vi "Vision_Processing_L_R10.vi"(0 "Current State":T1(ring)=enum."Normal - 5", 1 "Image Dst":T6=refnum, 2 "Inpute Image":T6=refnum, 3 "Startup Flag":bool, 5 "Current ROI Descriptor":T11={"Global Rectangle"=[22, 72, 300, 116], "Contours"=[{"ID"=enum."External", "Type"=12, "Coordinates"=[22, 72, 300, 116, 0]}]} {"Contours"."Type" items=["No Selection", "Point", "Line", "Rectangle", "Oval", "Polygon", "Freehand Region", "Annulus", "Unused2", "Unused3", "Broken Line", "Freehand Line", "Rotated Rectangle"]}, 6 "Avg Score - Last":dbl=954.6385864257812, 7 "error in (no error)":errorcluster, 8 "Current Settings":T9={"Curve Parameters"={"Extraction Mode"=1, "Edge Threshold"=150, "Edge Filter Size"=0, "Min Length"=15, "Row Search Step Size"=10, "Col Search Step Size"=10, "Max Endpoint Gap"=2, "Closed"=TRUE, "Subpixel"=TRUE}, "Match Mode"={"Rotation"=FALSE, "Scale"=TRUE, "Occlusion"=TRUE, "Reserved"=FALSE, "Reserved"=FALSE, "Reserved"=FALSE}, "Range Settings"=[{"Match Constraints"=0, "Min"=-2.0, "Max"=2.0}, {"Match Constraints"=1, "Min"=38.665856552124026, "Max"=79.77148170471192}, {"Match Constraints"=2, "Min"=0.0, "Max"=20.0}], "Number of Matches"=1, "Minimum Match Score"=879.6386, "SubPixel Accuracy"=TRUE, "Adv. Geometric Match Options 2"=[{"Setup Data Item"=20, "Item Value"=0.0}, {"Setup Data Item"=22, "Item Value"=1.0}]} {"Curve Parameters"."Extraction Mode" items=["Normal", "Uniform Regions"]; "Curve Parameters"."Edge Filter Size" items=["Fine", "Normal", "Contour Tracing"]; "Curve Parameters"."Max Endpoint Gap" min=0; "Curve Parameters"."Col Search Step Size" min=1 max=255 step=1; "Curve Parameters"."Row Search Step Size" min=1 max=255 step=1; "Curve Parameters"."Min Length" min=0; "Curve Parameters"."Edge Threshold" min=1 max=350 step=1; "Range Settings"."Max" format="%.2f"; "Range Settings"."Min" format="%.2f"; "Range Settings"."Match Constraints" items=["Rotation Angle (degrees)", "Scale Factor (%)", "Occlusion (%)"]; "Adv. Geometric Match Options 2"."Setup Data Item" items=["Curve Extraction Mode", "Curve Edge Threshold", "Curve Edge Filter Size", "Min Curve Length", "Curve Row Search Step Size", "Curve Col Search Step Size", "Curve Max Endpoint Gap", "Extract Closed Curves", "Enable Subpixel Curve Extraction", "Enable Correlation Score", "Enable Subpixel Accuracy", "Subpixel Iterations", "Subpixel Tolerance", "Initial Match List Length", "Enable Target Template Curve Score", "Min Match Separation Distance", "Min Match Separation Angle", "Min Match Separation Scale", "Max Match Overlap", "Enable Coarse Result", "Enable Calibration Support", "Enable Contrast Reversal", "Search Strategy", "Refinement Match Factor", "Subpixel Match Factor"]}, 9 "Sub Beacon Search Enable":bool[](array[boolean])=[FALSE, FALSE, FALSE, FALSE, FALSE], 10 "History Data - IN":T5={"Valid Beacon History - in"=[TRUE, TRUE, TRUE, TRUE, TRUE, TRUE, TRUE, TRUE, TRUE, TRUE, TRUE, TRUE, TRUE, TRUE, TRUE, TRUE, TRUE, TRUE, TRUE, TRUE], "Valid Score History"=[951.256103515625, 952.61669921875, 953.3775024414062, 959.8223266601562, 956.1203002929688, 952.1344604492188, 956.0997314453125, 948.7136840820312, 952.3104858398438, 956.33447265625, 949.6373291015625, 958.9732055664062, 951.8001708984375, 950.714599609375, 947.1436767578125, 952.746337890625, 992.2626342773438, 961.8504028320312, 971.9244384765625, 991.4178466796875], "Valid Scale History"=[59.26946258544922, 59.40597152709961, 59.318138122558594, 58.82406997680664, 59.27570343017578, 59.32193374633789, 59.52216339111328, 59.563385009765625, 59.49657440185547, 59.222198486328125, 59.44833755493164, 58.8350830078125, 59.57790756225586, 59.5397834777832, 59.55012512207031, 59.43376922607422, 59.040557861328125, 58.843505859375, 58.907012939453125, 58.86661911010742]} {"Valid Scale History" format="%#_13g"; "Valid Score History" format="%#_13g"}, 13 "Avg Scale - Last":dbl=59.21866912841797, 16 "History Size":i32=20) -> (11 "Avg Scale":dbl=59.21866912841797, 12 "Avg Score":dbl=954.6385864257812, 14 "Tracking Info 1":T2={"Tracking Coordinates"={"X"=160.85008239746094, "Y"=94.3125991821289}, "Current Valid"=TRUE, "Current State - Out"=enum."Normal - 5", "Setting Values"={"Min Scale"=38.67179412841797, "Max Scale"=79.78653259277344, "Min Score"=879.8142578125}}, 15 "Next Main ROI Descriptor":T3={"Global Rectangle"=[22, 72, 300, 116], "Contours"=[{"ID"=enum."External", "Type"=12, "Coordinates"=[22, 72, 300, 116, 0]}]} {"Contours"."Type" items=["No Selection", "Point", "Line", "Rectangle", "Oval", "Polygon", "Freehand Region", "Annulus", "Unused2", "Unused3", "Broken Line", "Freehand Line", "Rotated Rectangle"]}, 17 "Beacon - Scales":sgl[](array[numeric])=[0.0, 59.087868, 59.67315, 57.828133, 55.61106], 18 "History Data - Out":T4={"Valid Beacon History\nOut"=[TRUE, TRUE, TRUE, TRUE, TRUE, TRUE, TRUE, TRUE, TRUE, TRUE, TRUE, TRUE, TRUE, TRUE, TRUE, TRUE, TRUE, TRUE, TRUE, TRUE], "Valid Score History\nOut"=[951.256103515625, 952.61669921875, 953.3775024414062, 959.8223266601562, 956.1203002929688, 952.1344604492188, 956.0997314453125, 948.7136840820312, 952.3104858398438, 956.33447265625, 949.6373291015625, 958.9732055664062, 951.8001708984375, 950.714599609375, 947.1436767578125, 952.746337890625, 992.2626342773438, 961.8504028320312, 971.9244384765625, 991.4178466796875], "Valid Scale History\nOut"=[59.26946258544922, 59.40597152709961, 59.318138122558594, 58.82406997680664, 59.27570343017578, 59.32193374633789, 59.52216339111328, 59.563385009765625, 59.49657440185547, 59.222198486328125, 59.44833755493164, 58.8350830078125, 59.57790756225586, 59.5397834777832, 59.55012512207031, 59.43376922607422, 59.040557861328125, 58.843505859375, 58.907012939453125, 58.86661911010742]} {"Valid Scale History\nOut" format="%#_13g"; "Valid Score History\nOut" format="%#_13g"}, 19 "Y Coordinates":sgl[](array[numeric])=[0.0, 93.79849, 95.07948, 94.243286, 94.8068], 20 "Beacons Found":bool[](array[boolean])=[FALSE, TRUE, TRUE, TRUE, TRUE], 21 "X Coordinates":sgl[](array[numeric])=[0.0, 119.799255, 161.4642, 200.06786, 238.5652], 22 "Next State":T1(ring)=enum."Normal - 5", 23 "Lock Status":bool=TRUE, 24 "Startup Flag - out":bool, 25 "New Settings":T9={"Curve Parameters"={"Extraction Mode"=1, "Edge Threshold"=150, "Edge Filter Size"=0, "Min Length"=15, "Row Search Step Size"=10, "Col Search Step Size"=10, "Max Endpoint Gap"=2, "Closed"=TRUE, "Subpixel"=TRUE}, "Match Mode"={"Rotation"=FALSE, "Scale"=TRUE, "Occlusion"=TRUE, "Reserved"=FALSE, "Reserved"=FALSE, "Reserved"=FALSE}, "Range Settings"=[{"Match Constraints"=0, "Min"=-2.0, "Max"=2.0}, {"Match Constraints"=1, "Min"=38.665856552124026, "Max"=79.77148170471192}, {"Match Constraints"=2, "Min"=0.0, "Max"=20.0}], "Number of Matches"=1, "Minimum Match Score"=879.6386, "SubPixel Accuracy"=TRUE, "Adv. Geometric Match Options 2"=[{"Setup Data Item"=20, "Item Value"=0.0}, {"Setup Data Item"=22, "Item Value"=1.0}]} {"Curve Parameters"."Extraction Mode" items=["Normal", "Uniform Regions"]; "Curve Parameters"."Edge Filter Size" items=["Fine", "Normal", "Contour Tracing"]; "Curve Parameters"."Max Endpoint Gap" min=0; "Curve Parameters"."Col Search Step Size" min=1 max=255 step=1; "Curve Parameters"."Row Search Step Size" min=1 max=255 step=1; "Curve Parameters"."Min Length" min=0; "Curve Parameters"."Edge Threshold" min=1 max=350 step=1; "Range Settings"."Max" format="%.2f"; "Range Settings"."Min" format="%.2f"; "Range Settings"."Match Constraints" items=["Rotation Angle (degrees)", "Scale Factor (%)", "Occlusion (%)"]}, 27 "Right Image 2":T6(plugin-control))   [LabVIEW 2015]
uses:
  <vilib>/vision/Image Controls.llb/IMAQ Image.ctl
  <vilib>/vision/Pattern Matching.llb/IMAQ Curve Parameters.ctl
  <vilib>/vision/Pattern Matching.llb/IMAQ Match Range Setting.ctl
panel:
  in  "Current State 3":T1(ring)
  in  "Current State 2":T1(ring)
  in  "ROBOT STATE(fwd, bwd, neither)":i32
  out "beacon - Scores":sgl[](array[numeric])=[0.0, 997.01117, 999.39996, 999.517, 998.72253]
  in  "Minimum Score\nNormal 5":dbl=800.0
  in  "Minimum Score\nSub 4":dbl=850.0
  in  "Minimum Score\nSub 3":dbl=900.0
  in  "Minimum Score\nSub 2":dbl=950.0
  in  "Sub - 4 - FIle Path":path=path "/home/lvuser/natinst/bin/BeaconTemplates/4_beacons_left.png"
  in  "3 / 2\nTransition Scale":sgl=100.0
  in  "Score\nCushion- tight":dbl=75.0
  in  "Main ROI Decay\nper Fail (Vertical)":i32=5
  in  "ROI_factor(Horiztonal) (2 b)":sgl=1.5
  in  "ROI_factor(vertical) (2 b)":sgl=2.5
  in  "Sub - 2 File Path":path=path "/home/lvuser/natinst/bin/BeaconTemplates/2_beacons_left.png"
  out "Scale Decay \nFactor":dbl=20.552812576293945
  in  "Scale Decay \nFactor":dbl=5.0
  in  "Valid Treshold\nfor Lock":i16=3
  in  "Horiztonall Beacon \nCushion (pixels)":sgl=20.0
  out "New Min Score":dbl=879.6385864257812
  out "New Low Scale":dbl=38.665856552124026
  out "New high Scale":dbl=79.77148170471192
  in  "Absolute\nMinimum Score":dbl=800.0
  in  "Absolute\nMaximum Scale":dbl=300.0
  in  "Absolute\nMinimum Scale":dbl=10.0
  in  "Default No Lock\nSetting Values":T10={"Min Scale"=20.0, "Max Scale"=170.0, "Min Score"=800.0}
  in  "Score\nCushion":dbl=75.0
  out "Scale \nCushion":dbl=20.552812576293945
  in  "5 / 4\nTransition Scale":sgl=60.0
  in  "4 / 3\nTransition Scale":sgl=85.0
  in  "Timeout \nThrehsold":i32=1000
  in  "Main ROI Decay\nper Fail (Horiztonal)":i32=25
  in  "ROI_factor(Horiztonal) (4 b)":sgl=5.0
  in  "ROI_factor(vertical) (4 b)":sgl=1.5
  in  "ROI_factor(vertical) (5 b)":sgl=2.7
  in  "ROI_factor(Horiztonal) (5 b)":sgl=4.7
  out "Current  Score":sgl=951.2561
  out "Current  Scale":sgl=59.269463
  in  "Fail Count - In":i32
  in  "Sub Beacon Template File Path - ARRAY":path[](array[path])=[path "/home/lvuser/natinst/bin/BeaconTemplates/Sub1.png", path "/home/lvuser/natinst/bin/BeaconTemplates/Sub2.png", path "/home/lvuser/natinst/bin/BeaconTemplates/Sub3.png", path "/home/lvuser/natinst/bin/BeaconTemplates/Sub4.png", path "/home/lvuser/natinst/bin/BeaconTemplates/Sub5.png"]
  in  "Sub - 3 - FIle Path":path=path "/home/lvuser/natinst/bin/BeaconTemplates/3_beacons_left.png"
  in  "Normal - 5 - File Path":path=path "/home/lvuser/natinst/bin/BeaconTemplates/5_beacons.png"
  # "INPUTS"
  # "FILE PATHS"
  # "CONFIG"
  # "OUTPUTS"
  # "************"
  # "Range"
  # "Range"
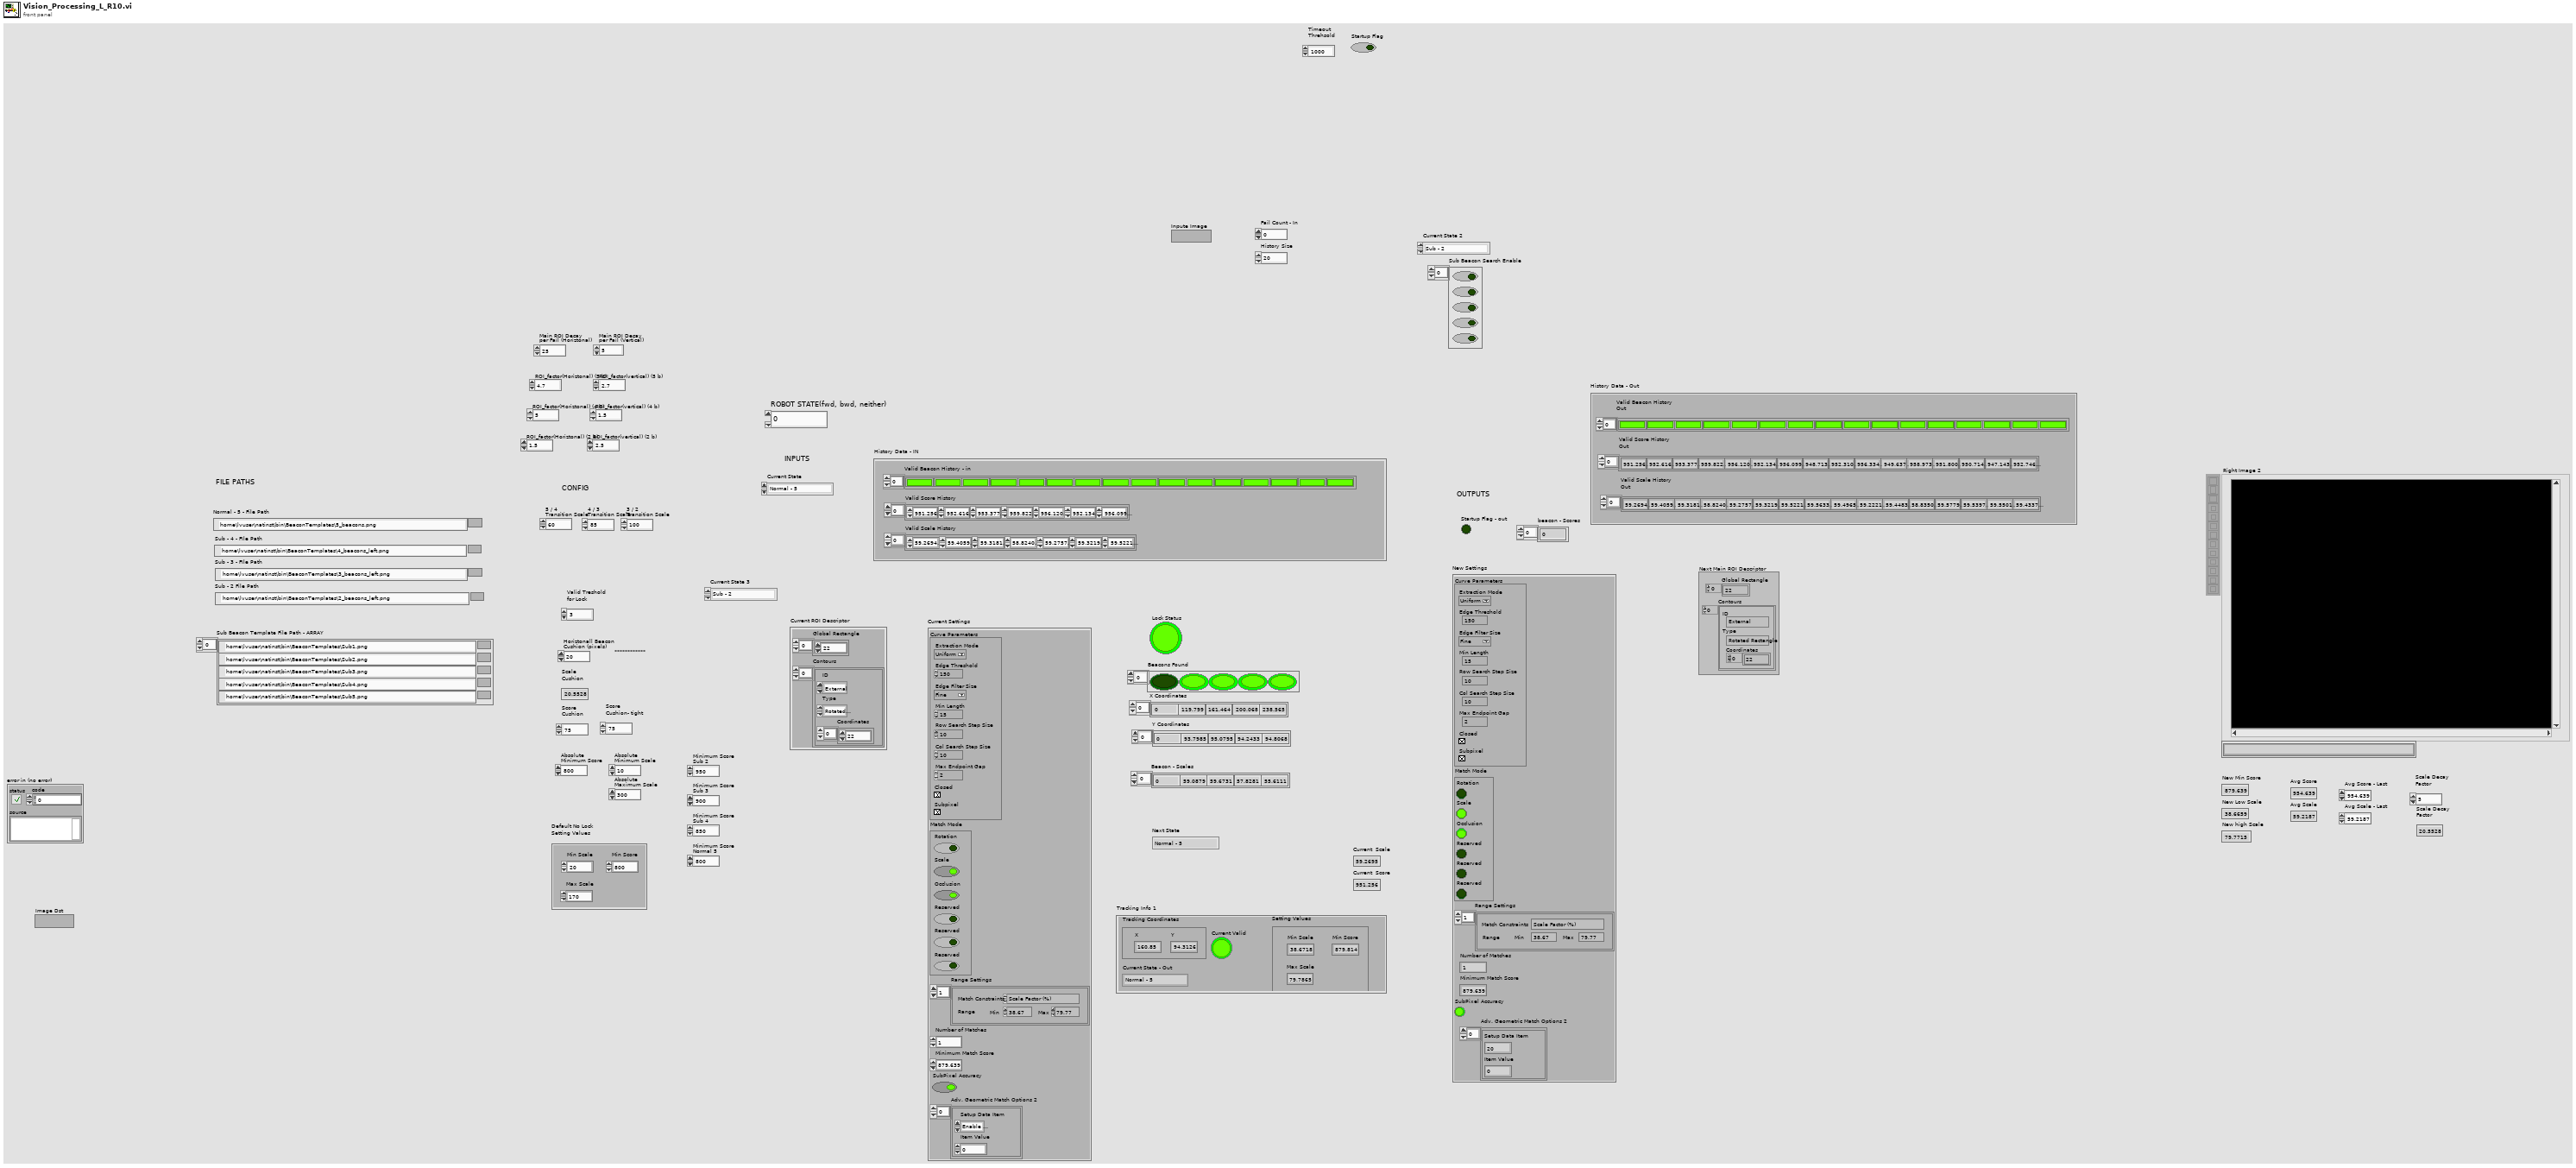
[diagram p1: front panel]
types:
  T1 = enum16{"Sub - 2", "Sub - 3", "Sub - 4", "Normal - 5"}
  T2 = cluster{"Tracking Coordinates":cluster{"X":dbl, "Y":dbl}, "Current Valid":bool, "Current State - Out":enum16{"Sub - 2", "Sub - 3", "Sub - 4", "Normal - 5"}, "Setting Values":cluster{"Min Scale":dbl, "Max Scale":dbl, "Min Score":dbl}}
  T3 = typedef "ROI Descriptor" = cluster{"Global Rectangle":i32[], "Contours":cluster{"ID":enum32{"External", "Internal"}, "Type":u32, "Coordinates":i32[]}[]}
  T4 = cluster{"Valid Beacon History\nOut":bool[], "Valid Score History\nOut":dbl[], "Valid Scale History\nOut":dbl[]}
  T5 = cluster{"Valid Beacon History - in":bool[], "Valid Score History":dbl[], "Valid Scale History":dbl[]}
  T6 = typedef "IMAQ Image.ctl" = refnum<image>
  T7 = typedef "IMAQ Curve Parameters.ctl" = cluster{"Extraction Mode":u32, "Edge Threshold":i32, "Edge Filter Size":u32, "Min Length":i32, "Row Search Step Size":i32, "Col Search Step Size":i32, "Max Endpoint Gap":i32, "Closed":bool, "Subpixel":bool}
  T8 = typedef "IMAQ Match Range Setting.ctl" = cluster{"Match Constraints":u32, "Min":dbl, "Max":dbl}
  T9 = cluster{"Curve Parameters":T7, "Match Mode":cluster{"Rotation":bool, "Scale":bool, "Occlusion":bool, "Reserved":bool, "Reserved":bool, "Reserved":bool}, "Range Settings":T8[], "Number of Matches":i32, "Minimum Match Score":sgl, "SubPixel Accuracy":bool, "Adv. Geometric Match Options 2":cluster{"Setup Data Item":u16, "Item Value":dbl}[]}
  T10 = cluster{"Min Scale":dbl, "Max Scale":dbl, "Min Score":dbl}
  T11 = cluster{"Global Rectangle":i32[], "Contours":cluster{"ID":enum32{"External", "Internal"}, "Type":u32, "Coordinates":i32[]}[]}
  T12 = typedef "IMAQ GM Match Report.ctl" = cluster{"Position":cluster{"x":sgl, "y":sgl}, "Angle":sgl, "Scale":sgl, "Score":sgl, "Bounding Box":cluster{"x":sgl, "y":sgl}[], "Contrast Reversed":bool, "Occlusion %":sgl, "Template Target Curve Score":sgl, "Target Template Curve Score":sgl, "Correlation Score":sgl}
  T13 = cluster{"Matches (Geometric Matching 1)[0]":T12, "Matches (Geometric Matching 1)[1]":T12, "Matches (Geometric Matching 1)[2]":T12, "Matches (Geometric Matching 1)[3]":T12, "Matches (Geometric Matching 1)[4]":T12, "Matches (Geometric Matching 1)[5]":T12, "Matches (Geometric Matching 1)[6]":T12, "Matches (Geometric Matching 1)[7]":T12, "Matches (Geometric Matching 1)[8]":T12}
  T14 = cluster{"Bounding Box[0]":cluster{"x":sgl, "y":sgl}, "Bounding Box[1]":cluster{"x":sgl, "y":sgl}, "Bounding Box[2]":cluster{"x":sgl, "y":sgl}, "Bounding Box[3]":cluster{"x":sgl, "y":sgl}, "Bounding Box[4]":cluster{"x":sgl, "y":sgl}, "Bounding Box[5]":cluster{"x":sgl, "y":sgl}, "Bounding Box[6]":cluster{"x":sgl, "y":sgl}, "Bounding Box[7]":cluster{"x":sgl, "y":sgl}, "Bounding Box[8]":cluster{"x":sgl, "y":sgl}}
  T15 = cluster{"index":u32, "Absolute\nMinimum Scale":dbl, "Absolute\nMaximum Scale":dbl}
  T16 = cluster{"New Low Scale":dbl, "New high Scale":dbl, "New Min Score":dbl}
  T17 = cluster{"Position":cluster{"x":sgl, "y":sgl}, bool, "Current State - Out":enum16{"Sub - 2", "Sub - 3", "Sub - 4", "Normal - 5"}, cluster{"New Low Scale":dbl, "New high Scale":dbl, "New Min Score":dbl}}
  T18 = cluster{"Position":cluster{"x":sgl, "y":sgl}, bool, "Current State":enum16{"Sub - 2", "Sub - 3", "Sub - 4", "Normal - 5"}, cluster{"New Low Scale":dbl, "New high Scale":dbl, "New Min Score":dbl}}
  T19 = typedef "IMAQ Rectangle" = cluster{"Left":i32, "Top":i32, "Right":i32, "Bottom":i32, "Rotation":dbl}
  T20 = cluster{"index":u32, "Min Scale":dbl, "Max Scale":dbl}
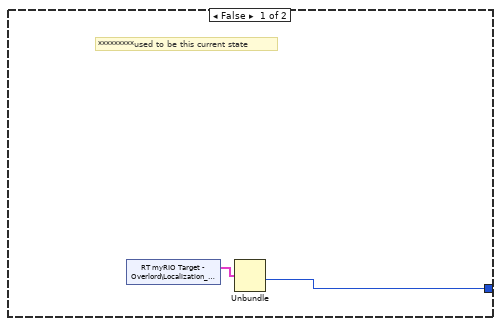
[diagram p4: hidden frame]
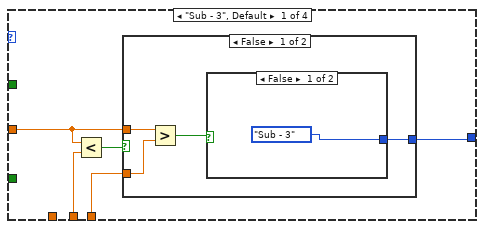
[diagram p5: hidden frame]
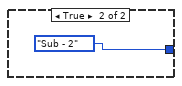
[diagram p6: hidden frame]
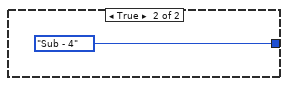
[diagram p7: hidden frame]
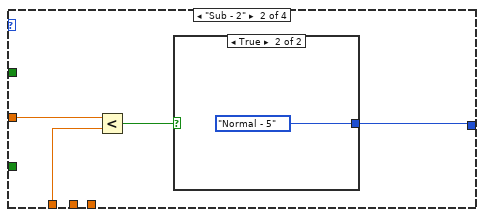
[diagram p8: hidden frame]
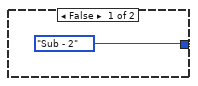
[diagram p9: hidden frame]
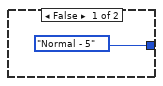
[diagram p10: hidden frame]
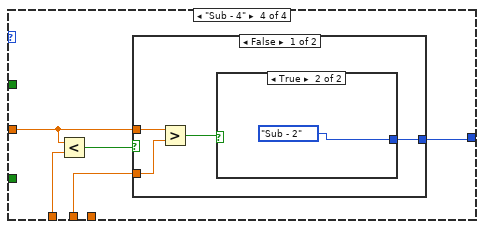
[diagram p11: hidden frame]
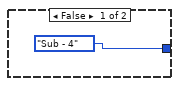
[diagram p12: hidden frame]
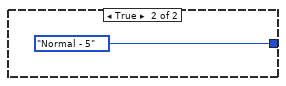
[diagram p13: hidden frame]
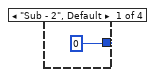
[diagram p15: hidden frame]
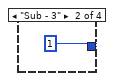
[diagram p16: hidden frame]
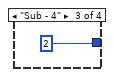
[diagram p17: hidden frame]
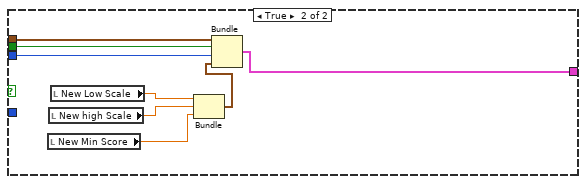
[diagram p18: hidden frame]
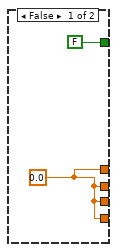
[diagram p19: hidden frame]
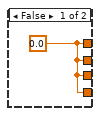
[diagram p20: hidden frame]
diagram:
  (unwired) enum16{"Short Range", "Long Range"}."Short Range"
  # "Next Settings"
  n1 = flat-sequence {
    tunnel: [w8] -> w3
    tunnel: [w7] -> w2
    tunnel: ["Image Dst"] -> w1
    tunnel: w3 -> [w159]
    tunnel: w2 -> [w157]
    tunnel: w1 -> [w158]
    frame #0 {
      # "APPLY FILTERING"
      n2 = call "Camera - Filtering"("Image In"="Inpute Image", "Image Dst"="Image Dst", "error in"="error in (no error)") -> ("Image Out"=w8:T6, "error out"=w7:errorcluster)  [unwired: 23 in]
    }
    frame #1 {
      w54 = u32 1 ("index")
      w123 = u32 1 ("index")
      w142 = u8 5
      # "*************************************************************************************************"
      # "Current Scale"
      # "Lower Scale"
      # "Upper Scale"
      # "Scale"
      # "Start up Template"
      # "Image Lock"
      # "Update Tracking Coordinates"
      # "CURRENT VALID"
      # "*************"
      # "Beacon - Y"
      # "Beacon - X"
      # "Beacons Found"
      # "Build ROI for Individual Beacons Based on Main Bounding Box"
      # "Starting X Lower Bound"
      # "Length of\nIndividual Beacon ROI"
      # "Length of Bounding Box"
      # "Choose ROI Factor based on Next State"
      # "Current Match"
      # "Current ROI"
      # "Image Lock"
      # "Force SR on Startup"
      # "Valid History"
      # "Draw ROI and stuff on outputi mage"
      # "Pull Down Startup IF Already True and Lock\nOtherwise don't update"
      # "Next Settings"
      # "Apply Limits to Settings"
      # "Scale"
      # "Min Score"
      # "Lower Scale"
      # "Upper Scale"
      # "Current Settings"
      # "Current Min\n& Max Scale"
      # "Current Valid"
      # "Update Search Settings"
      # "Update Template State"
      # "Calculate Average Scale/Score"
      # "max avg"
      # "Min Required to use avarage"
      # "Valid  Ccount\n(up to 3)"
      # "****# of previous in history that must be true\nin order for position to be considered \"locked\""
      # "Update Shift Arrays"
      # "# of Beacons Found to be valid"
      # "# of beacons"
      # "Matches"
      # "image out"
      n3 = Select(t=T1."Sub - 2", s="Startup Flag", f="Current State") -> (s? t:f=w62:T1)
      n4 = case shown="\"Sub - 2\"" w62 {
        tunnel: w159 -> [w539 w571 w602 w637]
        tunnel: w158 -> [w538 w570 w601 w636]
        tunnel: "Current ROI Descriptor" -> [w537 w569 w599 w635]
        tunnel: "Current Settings" -> [w536 w568 w598 w634]
        tunnel: [w532 w564 w595 w630] -> w88
        tunnel: [w531 w563 w596 w629] -> w108
        tunnel: [w529 w561 w597 w627] -> w150
        tunnel: w157 -> [_ _ w600 w626]
        tunnel: "Sub Beacon Search Enable" -> [w530 w562 w603 w625]
        tunnel: [sgl 3.0 ("y") sgl 2.0 ("y") 4.0 sgl 5.0 ("y")] -> w155
        tunnel: [w527 w559 w593 w623] -> w154
        tunnel: [2 1 3 4] -> w151
        frame "Sub - 3" {
          n5 = call "Short Range 2"("Image In"=w539, "Image Dst"=w538, "ROI Descriptor (Geometric Matching 1)"=w537, "Settings (Geometric Matching 1)"=w536, "Template File Path (Geometric Matching 1)"="Sub - 3 - FIle Path") -> ("Image Out"=w531:T6, "Matches (Geometric Matching 1)"=w532:T12[], "Number of Matches (Geometric Matching 1)"=w533:i32, "error out"=w527:errorcluster)  [unwired: 19 in]
          n6 = Equal?(x=w533, y=1) -> (x = y?=w534:bool)
          n7 = case shown="True" w534 {
            tunnel: w530 -> [w547 w550]
            tunnel: [w540 w551] -> w529
            frame False {
              w541 = FALSE
              # "F"
              # "No Main Found,\nDon't Search any Subs"
              n8 = Replace Array Subset(array=w547, new element #1=w541, index #1=0 ("y"), new element #2=w541, index #2=1 ("y"), new element #3=w541, index #3=2 ("y"), new element #4=w541, index #4=3 ("y"), new element #5=w541, index #5=4 ("y")) -> (w540:bool[])
            }
            frame True {
              w549 = TRUE
              w548 = FALSE
              n9 = Replace Array Subset(array=w550, new element #1=w549, index #1=0 ("y"), new element #2=w549, index #2=1 ("y"), new element #3=w549, index #3=2 ("y"), new element #4=w548, index #4=3 ("y"), new element #5=w548, index #5=4 ("y")) -> (w551:bool[])
            }
          }
        }
        frame "Sub - 2" {
          n10 = call "Short Range"("Image In"=w571, "Image Dst"=w570, "ROI Descriptor (Geometric Matching 1)"=w569, "Settings (Geometric Matching 1)"=w568, "Template File Path (Geometric Matching 1)"="Sub - 2 File Path") -> ("Image Out"=w563:T6, "Matches (Geometric Matching 1)"=w564:T12[], "Number of Matches (Geometric Matching 1)"=w565:i32, "error out"=w559:errorcluster)  [unwired: 19 in]
          n11 = Equal?(x=w565, y=1) -> (x = y?=w566:bool)
          n12 = case shown="True" w566 {
            tunnel: w562 -> [w579 w582]
            tunnel: [w572 w583] -> w561
            frame False {
              w573 = FALSE
              # "F"
              # "No Main Found,\nDon't Search any Subs"
              n13 = Replace Array Subset(array=w579, new element #1=w573, index #1=0 ("y"), new element #2=w573, index #2=1 ("y"), new element #3=w573, index #3=2 ("y"), new element #4=w573, index #4=3 ("y"), new element #5=w573, index #5=4 ("y")) -> (w572:bool[])
            }
            frame True {
              w581 = TRUE
              w580 = FALSE
              # "Search for specific Beacons"
              n14 = Replace Array Subset(array=w582, new element #1=w581, index #1=0 ("y"), new element #2=w581, index #2=1 ("y"), new element #3=w580, index #3=2 ("y"), new element #4=w580, index #4=3 ("y"), new element #5=w580, index #5=4 ("y")) -> (w583:bool[])
            }
          }
        }
        frame "Sub - 4" {
          # "**Make sure this selects the \nappropriate beacons to search for!!"
          n15 = call "Dumping Range"("Image In"=w602, "Image Dst"=w601, "ROI Descriptor (Geometric Matching 1)"=w599, "Settings (Geometric Matching 1)"=w598, "Template File Path (Geometric Matching 1)"="Sub - 4 - FIle Path", "error in"=w600) -> ("Image Out"=w596:T6, "Matches (Geometric Matching 1)"=w595:T12[], "Number of Matches (Geometric Matching 1)"=w592:i32, "error out"=w593:errorcluster)  [unwired: 18 in]
          n16 = Equal?(x=w592, y=1) -> (x = y?=w590:bool)
          n17 = case shown="True" w590 {
            tunnel: w603 -> [w612 w615]
            tunnel: [w605 w616] -> w597
            frame False {
              w606 = FALSE
              # "F"
              # "No Main Found,\nDon't Search any Subs"
              n18 = Replace Array Subset(array=w612, new element #1=w606, index #1=0 ("y"), new element #2=w606, index #2=1 ("y"), new element #3=w606, index #3=2 ("y"), new element #4=w606, index #4=3 ("y"), new element #5=w606, index #5=4 ("y")) -> (w605:bool[])
            }
            frame True {
              w614 = TRUE
              n19 = Replace Array Subset(array=w615, new element #1=w614, index #1=0 ("y"), new element #2=w614, index #2=1 ("y"), new element #3=w614, index #3=2 ("y"), new element #4=w614, index #4=3 ("y"), new element #5=FALSE, index #5=4 ("y")) -> (w616:bool[])
            }
          }
        }
        frame "Normal - 5" {
          n20 = call "Long Range"("Image In"=w637, "Image Dst"=w636, "ROI Descriptor (Geometric Matching 1)"=w635, "Settings (Geometric Matching 1)"=w634, "Template File Path (Geometric Matching 1)"="Normal - 5 - File Path", "error in"=w626) -> ("Image Out"=w629:T6, "Matches (Geometric Matching 1)"=w630:T12[], "Number of Matches (Geometric Matching 1)"=w632:i32, "error out"=w623:errorcluster)  [unwired: 18 in]
          n21 = Equal?(x=w632, y=1) -> (x = y?=w628:bool)
          n22 = case shown="True" w628 {
            tunnel: w625 -> [w645 w647]
            tunnel: [w638 w646] -> w627
            frame False {
              w639 = FALSE
              # "F"
              # "No Main Found,\nDon't Search any Subs"
              n23 = Replace Array Subset(array=w645, new element #1=w639, index #1=0 ("y"), new element #2=w639, index #2=1 ("y"), new element #3=w639, index #3=2 ("y"), new element #4=w639, index #4=3 ("y"), new element #5=w639, index #5=4 ("y")) -> (w638:bool[])
            }
            frame True {
              w648 = TRUE
              # "T"
              # "Search for ALL Beacons"
              n24 = Replace Array Subset(array=w647, new element #1=w648, index #1=0 ("y"), new element #2=w648, index #2=1 ("y"), new element #3=w648, index #3=2 ("y"), new element #4=w648, index #4=3 ("y"), new element #5=w648, index #5=4 ("y")) -> (w646:bool[])
            }
          }
        }
      }
      n25 = Array To Cluster(array=w88) -> (cluster=w86:T13)
      n26 = Unbundle By Name(w86) -> ("Matches (Geometric Matching 1)[0].Position"=w64:cluster{"x":sgl, "y":sgl}, "Matches (Geometric Matching 1)[0].Bounding Box"=w84:cluster{"x":sgl, "y":sgl}[], "Matches (Geometric Matching 1)[0].Scale"=w44:sgl, "Matches (Geometric Matching 1)[0].Score"=w115:sgl)
      "Current  Scale" <- w44
      "Current  Score" <- w115
      n27 = Array To Cluster(array=w84) -> (cluster=w85:T14)
      n28 = Unbundle By Name(w85) -> ("Bounding Box[0].x"=w75:sgl, "Bounding Box[0].y"=w74:sgl, "Bounding Box[2].x"=w73:sgl, "Bounding Box[2].y"=w72:sgl)
      n29 = Bundle("x"=w75, "y"=w74, "x"=w73, "y"=w72) -> (w70:cluster{"x":sgl, "y":sgl, "x":sgl, "y":sgl})  [unwired: 1 in]
      n30 = call "IMAQ Overlay Rectangle"("Rectangle"=w70, "Image"=w108) -> ("Image Out"=w71:T6)  [unwired: 8 in, 1 out]
      n31 = Subtract(x=w73, y=w75) -> (x-y=w79:sgl)
      n32 = Divide(x=w79, y=w155) -> (x/y=w81:dbl)
      n33 = Multiply(x="Horiztonall Beacon \nCushion (pixels)", y=w44) -> (x*y=w69:sgl)
      n34 = Divide(x=w69, y=sgl 100.0) -> (x/y=w66:sgl)
      n35 = Subtract(x=w74, y=w66) -> (x-y=w82:sgl)
      n36 = Add(x=w66, y=w72) -> (x+y=w83:sgl)
      n37 = for {
        N: 5 -> [_]
        tunnel: w150 -> [w305] mode=indexing
        shift-right: [w299] -> _
        shift-left: w75 -> [w304]
        tunnel: w81 -> [w303]
        tunnel: w82 -> [w296]
        tunnel: w83 -> [w295]
        tunnel: [w302] -> w77 mode=indexing
        tunnel: w66 -> [w297]
        # "Divide Bounding Box"
        # "Upper Bound of Current is\nLower Bound for Next"
        n38 = case shown="True" w305 {
          tunnel: w304 -> [w306 w307]
          tunnel: w303 -> [_ w309]
          tunnel: [w306 w308] -> w299
          tunnel: [w306 w307] -> w301
          frame False {
            # "Don't Care"
          }
          frame True {
            # "X Lower Bound"
            n39 = Add(x=w307, y=w309) -> (x+y=w308:dbl)
          }
        }
        n40 = Subtract(x=w301, y=w297) -> (x-y=w300:dbl)
        n41 = Add(x=w299, y=w297) -> (x+y=w298:dbl)
        n42 = call "Bound_RO_R_R0I.vi"("Bottom Right - Y"=w295, "Right - X"=w298, "Top Left - Y"=w296, "Top  Left - x"=w300) -> ("ROI Descriptor"=w302:T3)  [unwired: 7 in]
      }
      n43 = local read "Absolute\nMaximum Scale"() -> (w45:dbl)
      n44 = local read "Absolute\nMinimum Scale"() -> (w46:dbl)
      n45 = local read "Scale \nCushion"() -> (w43:dbl)
      n46 = Add(x=w44, y=w43) -> (x+y=w41:dbl)
      n47 = Subtract(x=w44, y=w43) -> (x-y=w42:dbl)
      n48 = Less?(x=w42, y=w46) -> (x < y?=w50:bool)
      n49 = Greater?(x=w41, y=w45) -> (0:w47:bool)
      n50 = Greater?(x=w42, y=w41) -> (0:w51:bool)
      n51 = Less?(x=w41, y=w42) -> (x < y?=w48:bool)
      n52 = Or(x=w50, y=w51) -> (x .or. y?=w52:bool)
      n53 = Or(x=w47, y=w48) -> (x .or. y?=w49:bool)
      n54 = Select(t=w46, s=w52, f=w42) -> (s? t:f=w40:dbl)
      n55 = Select(t=w45, s=w49, f=w41) -> (s? t:f=w39:dbl)
      n56 = Unbundle By Name("Current Settings") -> ("Range Settings"=w35:T8[])
      n57 = Bundle("index"=w54, "Absolute\nMinimum Scale"=w40, "Absolute\nMaximum Scale"=w39) -> (w53:T15)  [unwired: 1 in]
      n58 = Replace Array Subset(array=w35, new element=w53, index=w54) -> (w38:T8[])
      n59 = Bundle By Name(cluster="Current Settings", "Range Settings"=w38) -> (w37:T9)
      n60 = for {
        N: 5 -> [_]
        tunnel: w108 -> [w272]
        tunnel: w154 -> [w271]
        tunnel: w77 -> [w264] mode=indexing
        tunnel: "Sub Beacon Template File Path - ARRAY" -> [w270] mode=indexing
        tunnel: [w269] -> w57 mode=indexing
        tunnel: [w268] -> w56 mode=indexing
        tunnel: [w267] -> w58 mode=indexing
        tunnel: w150 -> [w266] mode=indexing
        tunnel: w37 -> [w265]
        shift-right: [w262] -> w109
        shift-left: w71 -> [w263]
        tunnel: [w261] -> w99 mode=indexing
        tunnel: [w260] -> w34 mode=indexing
        n61 = case shown="True" w266 {
          tunnel: w272 -> [_ w287]
          tunnel: w271 -> [_ w286]
          tunnel: w264 -> [_ w285]
          tunnel: w270 -> [_ w284]
          tunnel: [w273 w280] -> w269
          tunnel: [w273 w279] -> w268
          tunnel: [FALSE w278] -> w267
          tunnel: w265 -> [_ w277]
          tunnel: [w273 w276] -> w261
          tunnel: [w273 w275] -> w260
          frame False {
            w273 = sgl 0.0 ("x")
          }
          frame True {
            n62 = call "Sub Beacon Pattern Match"("Image In"=w287, "ROI Descriptor (Geometric Matching 1)"=w285, "Settings (Geometric Matching 1)"=w277, "Template File Path (Geometric Matching 1)"=w284, "error in"=w286) -> ("Matches (Geometric Matching 1)"=w281:T12[], "Number of Matches (Geometric Matching 1)"=w282:i32)  [unwired: 19 in, 2 out]
            n63 = Equal?(x=w282, y=1) -> (x = y?=w278:bool)
            n64 = case shown="True" w278 {
              tunnel: w281 -> [_ w293]
              tunnel: [w288 w292] -> w280
              tunnel: [w288 w291] -> w279
              tunnel: [w288 w290] -> w276
              tunnel: [w288 w289] -> w275
              frame False {
                w288 = sgl 0.0 ("x")
              }
              frame True {
                n65 = Array To Cluster(array=w293) -> (cluster=w294:T13)
                n66 = Unbundle By Name(w294) -> ("Matches (Geometric Matching 1)[0].Position.x"=w292:sgl, "Matches (Geometric Matching 1)[0].Position.y"=w291:sgl, "Matches (Geometric Matching 1)[0].Scale"=w290:sgl, "Matches (Geometric Matching 1)[0].Score"=w289:sgl)
              }
            }
          }
        }
        n67 = call "IMAQ Overlay ROI"("ROI Descriptor"=w264, "Image"=w263) -> ("Image Out"=w262:T6)  [unwired: 8 in, 1 out]
      }
      "Beacons Found" <- w58
      "X Coordinates" <- w57
      "Y Coordinates" <- w56
      "Beacon - Scales" <- w99
      "beacon - Scores" <- w34
      n68 = Boolean To (0,1)(Boolean=w58) -> (0, 1=w152:i16[])
      n69 = Add Array Elements(numeric array=w152) -> (sum=w153:i16)
      n70 = Greater Or Equal?(x=w153, y=w151) -> (x >= y?=w63:bool)
      n71 = case shown="False" w63 {
        tunnel: "Fail Count - In" -> [w523 _]
        tunnel: [w522 u16 0] -> w135
        frame False {
          n72 = Increment(x=w523) -> (x+1=w522:i32)
        }
        frame True {
          # "reset fail count"
        }
      }
      n73 = Unbundle By Name("History Data - IN") -> ("Valid Beacon History - in"=w106:bool[], "Valid Score History"=w105:dbl[], "Valid Scale History"=w104:dbl[])
      n74 = Greater?(x=w135, y="Timeout \nThrehsold") -> (0:w29:bool)
      n75 = Decrement(x="History Size") -> (x-1=w148:i32)
      n76 = for {
        N: "History Size" -> [_]
        shift-right: [w500] -> w103
        shift-left: w106 -> [w488]
        tunnel: w148 -> [w496]
        shift-right: [w493] -> w102
        shift-left: w105 -> [w495]
        shift-right: [w492] -> w101
        shift-left: w104 -> [w494]
        tunnel: w115 -> [w491]
        tunnel: w44 -> [w490]
        tunnel: w63 -> [w489]
        i -> [w499]
        # "Reverse Index"
        n77 = Subtract(x=w496, y=w499) -> (x-y=w497:i32)
        n78 = Equal To 0?(x=w497) -> (x = 0?=w498:bool)
        n79 = case shown="True" w498 {
          tunnel: w497 -> [w501 w520]
          tunnel: w488 -> [w511 w513]
          tunnel: [w509 w512] -> w500
          tunnel: w489 -> [_ w521]
          tunnel: w495 -> [w506 w519]
          tunnel: w494 -> [w505 w518]
          tunnel: [w504 w516] -> w493
          tunnel: [w503 w517] -> w492
          tunnel: w491 -> [_ w515]
          tunnel: w490 -> [_ w514]
          frame False {
            # "Shift Old"
            n80 = Decrement(x=w501) -> (x-1=w502:i32)
            n81 = Index Array(array=w511, index=w502) -> (element=w510:bool)
            n82 = Index Array(array=w506, index=w502) -> (element=w508:dbl)
            n83 = Index Array(array=w505, index=w502) -> (element=w507:dbl)
            n84 = Replace Array Subset(array=w511, new element=w510, index=w501) -> (w509:bool[])
            n85 = Replace Array Subset(array=w506, new element=w508, index=w501) -> (w504:dbl[])
            n86 = Replace Array Subset(array=w505, new element=w507, index=w501) -> (w503:dbl[])
          }
          frame True {
            # "Scale"
            # "Score"
            # "Valid"
            # "insert New"
            n87 = Replace Array Subset(array=w519, new element=w515, index=w520) -> (w516:dbl[])
            n88 = Replace Array Subset(array=w518, new element=w514, index=w520) -> (w517:dbl[])
            n89 = Replace Array Subset(array=w513, new element=w521, index=w520) -> (w512:bool[])
          }
        }
      }
      n90 = Boolean To (0,1)(Boolean=w103) -> (0, 1=w146:i16[])
      n91 = Bundle("Valid Beacon History - in"=w103, "Valid Score History"=w102, "Valid Scale History"=w101) -> (→"History Data - Out":T5)  [unwired: 1 in]
      n92 = Add Array Elements(numeric array=w146) -> (sum=w147:i16)
      n93 = Greater Or Equal?(x=w147, y="Valid Treshold\nfor Lock") -> (x >= y?=w30:bool)
      "Lock Status" <- w30
      n94 = Initialize Array(u8 0, w142) -> (w144:u8[])
      n95 = while {
        shift-right: [w471] -> w140
        shift-left: w144 -> [w473]
        tunnel: w103 -> [w479] mode=indexing
        shift-right: [w477] -> w138
        shift-left: u8 0 -> [w480]
        tunnel: "History Size" -> [w478]
        tunnel: w142 -> [w470]
        i -> [w472]
        stop <- w474 stop-if-true
        # "Grab Last 2 Valid Indexes"
        n96 = case shown="True" w479 {
          tunnel: w480 -> [w482 w484]
          tunnel: [w482 w487] -> w477
          tunnel: w473 -> [w481 w486]
          tunnel: w472 -> [_ w485]
          tunnel: [w481 w483] -> w471
          frame False {
          }
          frame True {
            # "Update Index\nto use"
            # "Increment\nValid Count"
            n97 = Replace Array Subset(array=w486, new element=w485, index=w484) -> (w483:u8[])
            n98 = Increment(x=w484) -> (x+1=w487:u8)
          }
        }
        n99 = Greater?(x=w472, y=w478) -> (0:w475:bool)
        n100 = Greater Or Equal?(x=w477, y=w470) -> (x >= y?=w476:bool)
        n101 = Or(x=w476, y=w475) -> (x .or. y?=w474:bool)
      }
      n102 = Greater?(x=w138, y=u8 2) -> (0:w139:bool)
      n103 = case shown="False" w139 {
        tunnel: w138 -> [_ w454]
        tunnel: w140 -> [_ w460]
        tunnel: w102 -> [_ w459]
        tunnel: w101 -> [_ w458]
        tunnel: ["Avg Score - Last" w452] -> w113
        tunnel: ["Avg Scale - Last" w451] -> w10
        frame False {
        }
        frame True {
          w457 = 0.0
          n104 = for {
            N: w454 -> [_]
            tunnel: w460 -> [w467] mode=indexing
            tunnel: w459 -> [w469]
            tunnel: w458 -> [w468]
            shift-right: [w465] -> w456
            shift-left: w457 -> [w463]
            shift-right: [w466] -> w455
            shift-left: w457 -> [w462]
            # "Fetch Last Valid Values"
            n105 = Index Array(array=w469, index=w467) -> (element=w464:dbl)
            n106 = Index Array(array=w468, index=w467) -> (element=w461:dbl)
            n107 = Add(x=w464, y=w463) -> (x+y=w465:dbl)
            n108 = Add(x=w461, y=w462) -> (x+y=w466:dbl)
          }
          n109 = To Double Precision Float(number=w454) -> (double precision float=w453:dbl)
          n110 = Divide(x=w456, y=w453) -> (x/y=w452:dbl)
          n111 = Divide(x=w455, y=w453) -> (x/y=w451:dbl)
        }
      }
      "Avg Score" <- w113
      "Avg Scale" <- w10
      n112 = case shown="True" w30 {
        tunnel: w29 -> [_ w177]
        tunnel: "4 / 3\nTransition Scale" -> [_ w176]
        tunnel: "5 / 4\nTransition Scale" -> [_ w175]
        tunnel: w10 -> [_ w174]
        tunnel: w30 -> [_ w173]
        tunnel: [w169 w172] -> w24
        tunnel: "3 / 2\nTransition Scale" -> [_ w171]
        frame False {
          # "*********used to be this current state"
          n113 = shared-variable "RT myRIO Target - Overlord\\Localization_Variables_r0.lvlib\\Info - Left"() -> (w170:T2)  [unwired: 1 in, 1 out]
          n114 = Unbundle(w170) -> ("Current State - Out"=w169:T1)  [unwired: 3 out]
        }
        frame True {
          # "Timeout"
          n115 = local read "Current State 3"() -> (w178:T1)
          n116 = case shown="\"Normal - 5\"" w178 {
            tunnel: w173 -> [_ _ _ _]
            tunnel: w174 -> [w182 w194 w199 w205]
            tunnel: w177 -> [_ _ _ _]
            tunnel: w176 -> [w183 _ _ w204]
            tunnel: w175 -> [_ w191 w198 w207]
            tunnel: [w179 w192 w197 w203] -> w172
            tunnel: w171 -> [w180 _ _ _]
            frame "Sub - 3", Default {
              n117 = Less?(x=w182, y=w183) -> (x < y?=w181:bool)
              n118 = case shown="False" w181 {
                tunnel: w182 -> [w187 _]
                tunnel: [w184 T1."Sub - 4"] -> w179
                tunnel: w180 -> [w186 _]
                frame False {
                  n119 = Greater?(x=w187, y=w186) -> (0:w185:bool)
                  n120 = case shown="False" w185 {
                    tunnel: [T1."Sub - 3" T1."Sub - 2"] -> w184
                    frame False {
                    }
                    frame True {
                    }
                  }
                }
                frame True {
                }
              }
            }
            frame "Sub - 2" {
              n121 = Less?(x=w194, y=w191) -> (x < y?=w193:bool)
              n122 = case shown="True" w193 {
                tunnel: [T1."Sub - 2" T1."Normal - 5"] -> w192
                frame False {
                }
                frame True {
                }
              }
            }
            frame "Normal - 5" {
              # "If Out of Scale Range\nor Timeout"
              n123 = Greater?(x=w199, y=w198) -> (0:w200:bool)
              n124 = case shown="True" w200 {
                tunnel: [T1."Normal - 5" T1."Sub - 2"] -> w197
                frame False {
                }
                frame True {
                }
              }
            }
            frame "Sub - 4" {
              n125 = Less?(x=w205, y=w207) -> (x < y?=w206:bool)
              n126 = case shown="False" w206 {
                tunnel: w205 -> [w211 _]
                tunnel: [w208 T1."Normal - 5"] -> w203
                tunnel: w204 -> [w210 _]
                frame False {
                  n127 = Greater?(x=w211, y=w210) -> (0:w209:bool)
                  n128 = case shown="True" w209 {
                    tunnel: [T1."Sub - 4" T1."Sub - 2"] -> w208
                    frame False {
                    }
                    frame True {
                    }
                  }
                }
                frame True {
                }
              }
            }
          }
        }
      }
      "Next State" <- w24
      n129 = local read "Current State"() -> (w59:T1)
      n130 = Equal?(x=w59, y=w24) -> (x = y?=w55:bool)
      n131 = case shown="False" w55 {
        tunnel: w64 -> [w224 w259]
        tunnel: w63 -> [w221 w258]
        tunnel: w62 -> [_ w257]
        tunnel: [w220 w256] -> w33
        tunnel: w24 -> [w218 _]
        tunnel: w58 -> [w228 _]
        tunnel: w57 -> [w226 _]
        tunnel: w56 -> [w225 _]
        frame False {
          # "Beacon Index"
          # "Check if Tracking is Available for the Next Template State"
          n132 = case shown="\"Normal - 5\"" w218 {
            tunnel: [0 1 2 1] -> w223
            frame "Sub - 2", Default {
            }
            frame "Sub - 3" {
            }
            frame "Sub - 4" {
            }
            frame "Normal - 5" {
            }
          }
          n133 = Index Array(array=w228, index=w223) -> (element=w227:bool)
          n134 = case shown="True" w227 {
            tunnel: w226 -> [_ w247]
            tunnel: w225 -> [_ w246]
            tunnel: [w229 w243] -> w222
            tunnel: w224 -> [w229 w244]
            tunnel: w223 -> [_ w245]
            frame False {
            }
            frame True {
              w240 = sgl 0.4 ("y")
              n135 = Unbundle(w244) -> ("x"=w241:sgl, "y"=w239:sgl)
              n136 = Index Array(array=w247, index=w245) -> (element=w236:sgl)
              n137 = Index Array(array=w246, index=w245) -> (element=w237:sgl)
              n138 = Subtract(x=sgl 1.0, y=w240) -> (x-y=w238:sgl)
              n139 = Multiply(x=w238, y=w236) -> (x*y=w234:sgl)
              n140 = Multiply(x=w238, y=w237) -> (x*y=w232:sgl)
              n141 = Multiply(x=w240, y=w241) -> (x*y=w235:sgl)
              n142 = Multiply(x=w240, y=w239) -> (x*y=w233:sgl)
              n143 = Add(x=w235, y=w234) -> (x+y=w231:sgl)
              n144 = Add(x=w233, y=w232) -> (x+y=w230:sgl)
              n145 = Bundle(w231, w230) -> (w243:cluster{sgl, sgl})  [unwired: 1 in]
            }
          }
          n146 = local read "New Min Score"() -> (w215:dbl)
          n147 = local read "New high Scale"() -> (w216:dbl)
          n148 = local read "New Low Scale"() -> (w217:dbl)
          n149 = Bundle("New Low Scale"=w217, "New high Scale"=w216, "New Min Score"=w215) -> (w219:T16)  [unwired: 1 in]
          n150 = Bundle("Position"=w222, w221, "Current State - Out"=w218, w219) -> (w220:T17)  [unwired: 1 in]
        }
        frame True {
          n151 = local read "New Min Score"() -> (w253:dbl)
          n152 = local read "New high Scale"() -> (w254:dbl)
          n153 = local read "New Low Scale"() -> (w255:dbl)
          n154 = Bundle("New Low Scale"=w255, "New high Scale"=w254, "New Min Score"=w253) -> (w252:T16)  [unwired: 1 in]
          n155 = Bundle("Position"=w259, w258, "Current State"=w257, w252) -> (w256:T18)  [unwired: 1 in]
        }
      }
      "Tracking Info 1" <- w33
      n156 = Unbundle By Name("Current Settings") -> ("Minimum Match Score"=w134:sgl, "Range Settings"=w120:T8[])
      n157 = case shown="\"Normal - 5\"" w24 {
        tunnel: "ROI_factor(vertical) (5 b)" -> [_ _ w168]
        tunnel: "ROI_factor(Horiztonal) (5 b)" -> [_ _ w167]
        tunnel: "ROI_factor(vertical) (4 b)" -> [_ w165 _]
        tunnel: "ROI_factor(Horiztonal) (4 b)" -> [_ w164 _]
        tunnel: "ROI_factor(vertical) (2 b)" -> [w162 _ _]
        tunnel: "ROI_factor(Horiztonal) (2 b)" -> [w161 _ _]
        tunnel: [w162 w165 w168] -> w14
        tunnel: [w161 w164 w167] -> w13
        tunnel: "Minimum Score\nSub 2" -> [w160 _ _]
        tunnel: [w160 w163 w166] -> w12
        tunnel: "Minimum Score\nNormal 5" -> [_ _ w166]
        tunnel: "Minimum Score\nSub 4" -> [_ w163 _]
        frame "Sub - 2" {
        }
        frame "Sub - 4", Default {
        }
        frame "Normal - 5" {
        }
      }
      n158 = Index Array(array=w120, index=u32 1) -> (element=w133:T8)
      n159 = Unbundle(w133) -> ("Min"=w131:dbl, "Max"=w130:dbl)  [unwired: 1 out]
      n160 = And(x="Startup Flag", y=w30) -> (x .and. y?=w118:bool)
      n161 = case shown="True" w118 {
        tunnel: "Startup Flag" -> [w310 _]
        tunnel: [w310 FALSE] -> w117
        frame False {
        }
        frame True {
        }
      }
      "Startup Flag - out" <- w117
      n162 = call "Scaling and Mapping2"("Signals"=w10) -> ("Scaled Signals"=w25:dynamicdata)  [unwired: 9 in, 1 out]
      n163 = To Single Precision Float(number=w25) -> (single precision float=w31:sgl)
      "Scale \nCushion" <- w31
      "Scale Decay \nFactor" <- w31
      n164 = call "Scaling and Mapping3"("Signals"=w10) -> ("Scaled Signals"=w9:dynamicdata)  [unwired: 9 in, 1 out]
      n165 = To Single Precision Float(number=w9) -> (single precision float=w11:sgl)
      n166 = case shown="True" w30 {
        tunnel: w63 -> [_ w370]
        tunnel: w113 -> [w324 w369]
        tunnel: w10 -> [w323 w368]
        tunnel: w134 -> [_ w367]
        tunnel: w131 -> [_ w366]
        tunnel: w130 -> [_ w365]
        tunnel: [w314 w344] -> w121
        tunnel: [w312 w356] -> w92
        tunnel: [w313 w355] -> w93
        tunnel: w31 -> [w326 w364]
        tunnel: "Score\nCushion" -> [w325 w363]
        tunnel: "Scale Decay \nFactor" -> [_ w362]
        tunnel: w31 -> [_ w361]
        tunnel: "Current ROI Descriptor" -> [_ w357]
        tunnel: w88 -> [_ w358]
        tunnel: w14 -> [_ w360]
        tunnel: w13 -> [_ w359]
        tunnel: [w316 w354] -> w87
        tunnel: w55 -> [_ w349]
        tunnel: w24 -> [_ w348]
        tunnel: w12 -> [_ w345]
        tunnel: "ROBOT STATE(fwd, bwd, neither)" -> [_ w343]
        tunnel: w11 -> [_ w342]
        frame False {
          # "Check Lock Status of OTHER Cam,\n\nif True,\n\nthen use it's settings,\n\notherwise use default no lock"
          # "Initial ROI Descriptor"
          # "Apply No Lock Default for each Template"
          n167 = disable-structure shown="Disabled" {
            disable-tunnel: [w341 _] -> _
            disable-tunnel: [w340 _] -> _
            disable-tunnel: w326 -> [w339 _]
            disable-tunnel: w325 -> [w338 _]
            disable-tunnel: w324 -> [w337 _]
            disable-tunnel: w323 -> [w336 _]
            frame Disabled {
              n168 = Subtract(x=w337, y=w338) -> ()  [unwired: 1 out]
              n169 = Subtract(x=w336, y=w339) -> (x-y=w341:dbl)
              n170 = Add(x=w339, y=w336) -> (x+y=w340:dbl)
            }
            frame Enabled {
            }
          }
          n171 = shared-variable "RT myRIO Target - Overlord\\Localization_Variables_r0.lvlib\\Image Lock - R"() -> (w315:bool)  [unwired: 1 in, 1 out]
          n172 = case shown="True" w315 {
            tunnel: [w329 w333] -> w314
            tunnel: [w327 w332] -> w313
            tunnel: [w328 w331] -> w312
            frame False {
              n173 = Unbundle By Name("Default No Lock\nSetting Values") -> ("Min Score"=w329:dbl, "Min Scale"=w328:dbl, "Max Scale"=w327:dbl)
            }
            frame True {
              n174 = shared-variable "RT myRIO Target - Overlord\\Localization_Variables_r0.lvlib\\Info - Right"() -> (w335:T2)  [unwired: 1 in, 1 out]
              n175 = Unbundle(w335) -> ("Setting Values"=w334:T10)  [unwired: 3 out]
              n176 = Unbundle(w334) -> ("Min Scale"=w331:dbl, "Max Scale"=w332:dbl, "Min Score"=w333:dbl)
            }
          }
          n177 = Bundle(0, 0, 640, 480, 0) -> (w322:cluster{i32, i32, i32, i32, i32})  [unwired: 1 in]
          n178 = call "IMAQ Convert Rectangle to ROI"("Rectangle"=w322) -> ("ROI Descriptor"=w316:T3)  [unwired: 8 in, 1 out]
        }
        frame True {
          # "Score out"
          # "Apply Limits to ROI"
          n179 = case shown="False" w370 {
            tunnel: w369 -> [_ w420]
            tunnel: [w388 w417] -> w346
            tunnel: w368 -> [_ w419]
            tunnel: [w387 w399] -> w356
            tunnel: [w386 w398] -> w355
            tunnel: w366 -> [w393 _]
            tunnel: w365 -> [w392 _]
            tunnel: w367 -> [w391 _]
            tunnel: w364 -> [_ w401]
            tunnel: w363 -> [_ w418]
            tunnel: w362 -> [w390 _]
            tunnel: w361 -> [w389 _]
            tunnel: w360 -> [_ w408]
            tunnel: w359 -> [_ w407]
            tunnel: w358 -> [_ w406]
            tunnel: [w379 w397] -> w353
            tunnel: [w378 w405] -> w352
            tunnel: [w377 w396] -> w351
            tunnel: [w376 w404] -> w350
            tunnel: w357 -> [w384 _]
            tunnel: w349 -> [_ _]
            tunnel: w348 -> [_ w403]
            tunnel: w343 -> [_ w394]
            tunnel: w342 -> [w372 _]
            frame False {
              # "Decrement Score by"
              n180 = Subtract(x=w393, y=w389) -> (x-y=w387:dbl)
              n181 = Add(x=w389, y=w392) -> (x+y=w386:dbl)
              n182 = Subtract(x=w391, y=w390) -> (x-y=w388:dbl)
              n183 = call "IMAQ Convert ROI to Rectangle"("ROI Descriptor"=w384) -> ("Rectangle"=w385:T19)  [unwired: 8 in, 1 out]
              n184 = Unbundle By Name(w385) -> ("Left"=w383:i32, "Top"=w382:i32, "Right"=w381:i32, "Bottom"=w380:i32)
              n185 = Divide(x=w372, y=sgl 10.0) -> (x/y=w371:sgl)
              n186 = To Long Integer(number=w372) -> (32bit integer=w374:i32)
              n187 = To Long Integer(number=w371) -> (32bit integer=w375:i32)
              n188 = Subtract(x=w383, y=w374) -> (x-y=w379:i32)
              n189 = Add(x=w381, y=w374) -> (x+y=w377:i32)
              n190 = Add(x=w380, y=w375) -> (x+y=w376:i32)
              n191 = Subtract(x=w382, y=w375) -> (x-y=w378:i32)
            }
            frame True {
              # "****"
              # "if switching states"
              # "Scale / Score"
              # "Main ROI"
              # "Horizontal Scale \n(smaller number = smaller ROI)"
              n192 = case shown="-1" w394 {
                tunnel: w419 -> [w424 w429 w434]
                tunnel: [w423 w425 w430] -> w402
                tunnel: w401 -> [w422 w428 w433]
                tunnel: [w421 w426 w431] -> w400
                frame 0, Default {
                  n193 = Subtract(x=w424, y=w422) -> (x-y=w421:dbl)
                  n194 = Add(x=w422, y=w424) -> (x+y=w423:dbl)
                }
                frame 1 {
                  n195 = Subtract(x=w429, y=5.0) -> (x-y=w426:dbl)
                  n196 = Add(x=w428, y=w429) -> (x+y=w425:dbl)
                }
                frame -1 {
                  n197 = Subtract(x=w434, y=w433) -> (x-y=w431:dbl)
                  n198 = Add(x=5.0 ("y"), y=w434) -> (x+y=w430:dbl)
                }
              }
              n199 = Subtract(x=w420, y=w418) -> (x-y=w417:dbl)
              n200 = Array To Cluster(array=w406) -> (cluster=w416:T13)
              n201 = Unbundle By Name(w416) -> ("Matches (Geometric Matching 1)[0].Position.x"=w410:sgl, "Matches (Geometric Matching 1)[0].Position.y"=w412:sgl, "Matches (Geometric Matching 1)[0].Scale"=w411:sgl)
              n202 = Divide(x=w411, y=w408) -> (x/y=w413:sgl)
              n203 = Multiply(x=w411, y=w407) -> (x*y=w415:sgl)
              n204 = Divide(x=w415, y=sgl 2.0) -> (x/y=w409:sgl)
              n205 = Add(x=w412, y=w413) -> (x+y=w404:sgl)
              n206 = Subtract(x=w412, y=w413) -> (x-y=w405:sgl)
              n207 = Subtract(x=w410, y=w409) -> (x-y=w397:sgl)
              n208 = Add(x=w409, y=w410) -> (x+y=w396:sgl)
              n209 = case shown="False" FALSE {
                tunnel: w403 -> [_ _]
                tunnel: [w437 w446] -> w398
                tunnel: w402 -> [w437 w448]
                tunnel: [w438 w445] -> w399
                tunnel: w400 -> [w438 w447]
                tunnel: w401 -> [_ w444]
                tunnel: [w436 w441] -> _
                tunnel: w397 -> [w436 w442]
                tunnel: [w435 w440] -> _
                tunnel: w396 -> [w435 w443]
                frame False {
                }
                frame True {
                  w439 = sgl 50.0 ("y")
                  # "Double scale cushion\nif changing states"
                  n210 = Add(x=w448, y=w444) -> (x+y=w446:dbl)
                  n211 = Subtract(x=w447, y=w444) -> (x-y=w445:dbl)
                  n212 = Subtract(x=w442, y=w439) -> (x-y=w441:sgl)
                  n213 = Add(x=w439, y=w443) -> (x+y=w440:sgl)
                }
              }
            }
          }
          n214 = Greater?(x=w346, y=w345) -> (0:w347:bool)
          n215 = call "Bound_RO_R_R0I.vi"("Bottom Right - Y"=w350, "Right - X"=w351, "Top Left - Y"=w352, "Top  Left - x"=w353) -> ("ROI Descriptor"=w354:T3)  [unwired: 7 in]
          n216 = Select(t=w346, s=w347, f=w345) -> (s? t:f=w344:dbl)
        }
      }
      "Next Main ROI Descriptor" <- w87
      n217 = Less?(x=w121, y="Absolute\nMinimum Score") -> (x < y?=w125:bool)
      n218 = Less?(x=w92, y="Absolute\nMinimum Scale") -> (x < y?=w95:bool)
      n219 = Greater?(x=w93, y="Absolute\nMaximum Scale") -> (0:w90:bool)
      n220 = Greater?(x=w92, y=w93) -> (0:w96:bool)
      n221 = Less?(x=w93, y=w92) -> (x < y?=w91:bool)
      n222 = Select(t="Absolute\nMinimum Score", s=w125, f=w121) -> (s? t:f=w127:dbl)
      "New Min Score" <- w127
      n223 = Or(x=w95, y=w96) -> (x .or. y?=w97:bool)
      n224 = Or(x=w90, y=w91) -> (x .or. y?=w94:bool)
      n225 = Select(t="Absolute\nMinimum Scale", s=w97, f=w92) -> (s? t:f=w110:dbl)
      "New Low Scale" <- w110
      n226 = Select(t="Absolute\nMaximum Scale", s=w94, f=w93) -> (s? t:f=w111:dbl)
      "New high Scale" <- w111
      n227 = Bundle("index"=w123, "Min Scale"=w110, "Max Scale"=w111) -> (w122:T20)  [unwired: 1 in]
      n228 = Replace Array Subset(array=w120, new element=w122, index=w123) -> (w124:T8[])
      n229 = call "IMAQ Overlay ROI"("ROI Descriptor"=w87, "Image"=w109) -> ("Image Out"=→"Right Image 2":T6)  [unwired: 8 in, 1 out]
      n230 = Bundle By Name(cluster="Current Settings", "Range Settings"=w124, "Minimum Match Score"=w127) -> (→"New Settings":T9)
    }
  }
